vi "PythonNode_AppendToIntegerArray.vi"() -> ()   [LabVIEW 2023]
doc: "This example demonstrates how to call a Python function and pass LabVIEW arrays as arguments. It uses a python function to append an element to an array of integers."
uses:
  support/PythonVersionsEnum.ctl
panel:
  out "modified array":i32[](array[numeric])
  in  "new element":i32=4
  in  "array":i32[](array[numeric])=[1, 2, 3]
  out "error out":errorcluster
  in  "error in (no error)":errorcluster
  in  "python version":T1
  # "Overview: Demonstrates how to call a Python function and pass arrays as arguments.\nRequirements: Python 3.6, 3.7, 3.8, 3.9 or 3.10 with the same bitness as LabVIEW.\nInstructions:\n1. Set the Python version to the version of Python you want to execute code in.\n2. Run the VI. You should see the result of appending \"new element\" to \"array\" in the indicator\n\"modified array\".\n3. See comments on the block diagram of this VI and in \"ExamplePythonModule.py\" for more information about how the call python node passes arguments and handles return values."
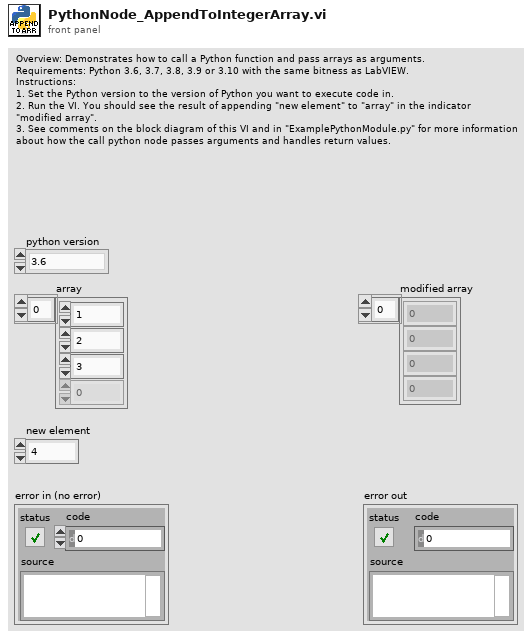
[diagram p1: front panel]
types:
  T1 = typedef "PythonVersionsEnum.ctl" = enum16{"3.6", "3.7", "3.8", "3.9", "3.10"}
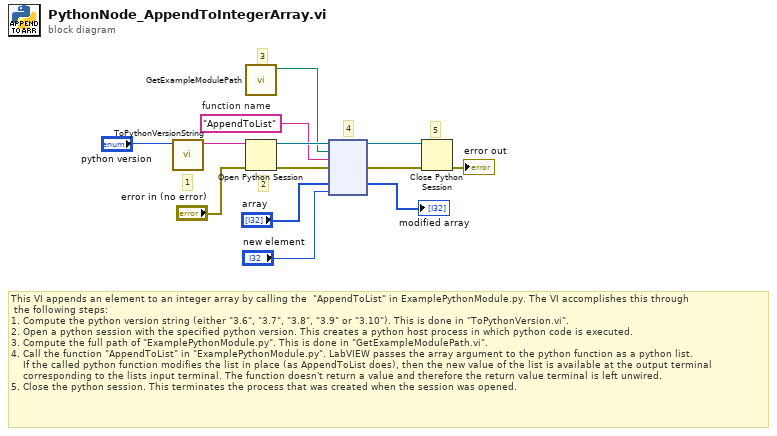
[diagram p0: block diagram]
diagram:
  w7 = "AppendToList"  # function name
  # "5"
  # "4"
  # "2"
  # "3"
  # "1"
  # "This VI appends an element to an integer array by calling the  \"AppendToList\" in ExamplePythonModule.py. The VI accomplishes this through\n the following steps:\n1. Compute the python version string (either \"3.6\", \"3.7\", \"3.8\", \"3.9\" or \"3.10\"). This is done in \"ToPythonVersion.vi\". \n2. Open a python session with the specified python version. This creates a python host process in which python code is executed.\n3. Compute the full path of \"ExamplePythonModule.py\". This is done in \"GetExampleModulePath.vi\".\n4. Call the function \"AppendToList\" in \"ExamplePythonModule.py\". LabVIEW passes the array argument to the python function as a python list.\n    If the called python function modifies the list in place (as AppendToList does), then the new value of the list is available at the output terminal\n    corresponding to the lists input terminal. The function doesn't return a value and therefore the return value terminal is left unwired.\n5. Close the python session. This terminates the process that was created when the session was opened."
  n1 = call "ToPythonVersionString.vi"("python version"="python version") -> ("python version string"=w13:string)  [unwired: 10 in]
  n2 = call "GetExampleModulePath.vi"() -> ("module path"=w8:path)  [unwired: 11 in]
  n3 = Open Python Session(python version=w13, 3:"error in (no error)") -> (session out=w10:refnum<k35>, error out=w9:errorcluster)  [unwired: 1 in]
  n4 = node(w10, w8, w7, w9, "array", "new element") -> (w6:refnum<k35>, w5:errorcluster, →"modified array":i32[])  [unwired: 3 in, 2 out]
  n5 = Close Python Session(session in=w6, error in=w5) -> (11:→"error out":errorcluster)
